vi "Define Advanced Sequence.vi"(4 "Current Level Start":dbl, 5 "name":string, 6 "Current Level Stop":dbl, 7 "Voltage Level Stop":dbl, 8 "error in (no error)":errorcluster, 9 "Points per Output Function":i32, 10 "Voltage Level Start":dbl, 11 "IVI Refnum in":refnum<k15>) -> (0 "error out":errorcluster, 1 "sequence name":string, 2 "Numeric":i32, 3 "IVI Refnum out":refnum<k15>)   [LabVIEW 2020]
uses:
  <instrlib>/niDCPower/nidcpower.llb/niDCPower Sequence Attribute Type.ctl
  <instrlib>/niDCPower/nidcpower.llb/niDCPower Output Function.ctl
  <instrlib>/niDCPower/nidcpower.llb/niDCPower Create Advanced Sequence Step With Channels.vi
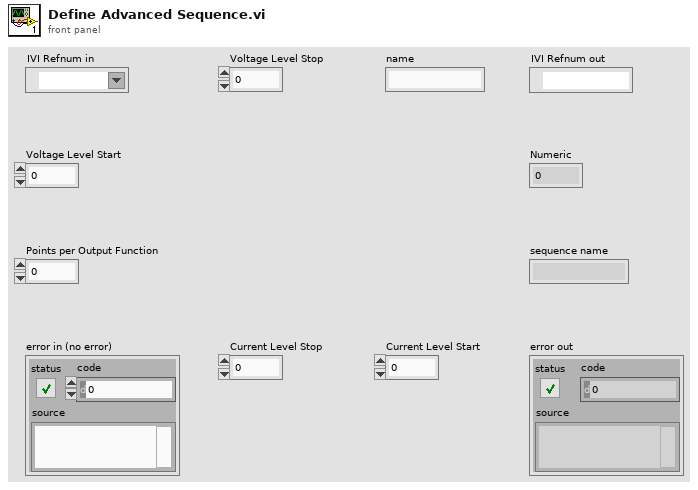
[diagram p1: front panel]
types:
  T1 = typedef "niDCPower Sequence Attribute Type.ctl" = i32
  T2 = typedef "niDCPower Output Function.ctl" = i32
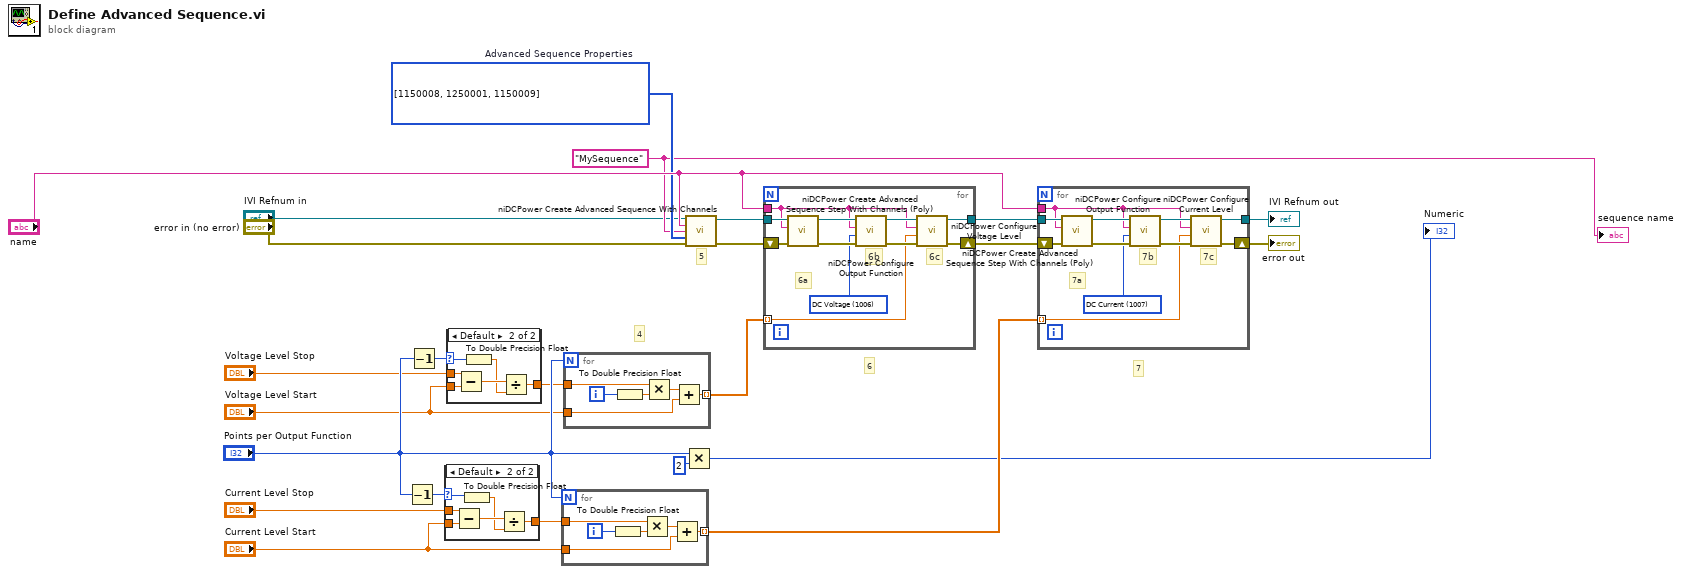
[diagram p0: block diagram]
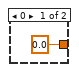
[diagram p2: hidden frame]
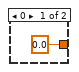
[diagram p3: hidden frame]
diagram:
  w23 = T1[] [1150008, 1250001, 1150009] items=["Source -> Output Function"=1150008, "Source -> Output Enabled"=1250006, "Source -> Output Resistance"=1150061, "Source -> Transient Response"=1150062, "Source -> Custom Transient Response -> Voltage Gain Bandwidth"=1150067, "Source -> Custom Transient Response -> Voltage Compensation Frequency"=1150068, "Source -> Custom Transient Response -> Voltage Pole-Zero Ratio"=1150069, "Source -> Custom Transient Response -> Current Gain Bandwidth"=1150070, "Source -> Custom Transient Response -> Current Compensation Frequency"=1150071, "Source -> Custom Transient Response -> Current Pole-Zero Ratio"=1150072, "Source -> DC Voltage -> Voltage Level"=1250001, "Source -> DC Voltage -> Voltage Level Range"=1150005, "Source -> DC Voltage -> Current Limit"=1250005, "Source -> DC Voltage -> Current Limit High"=1150187, "Source -> DC Voltage -> Current Limit Low"=1150188, "Source -> DC Voltage -> Current Limit Range"=1150004, "Source -> DC Current -> Current Level"=1150009, "Source -> DC Current -> Current Level Range"=1150011, "Source -> DC Current -> Voltage Limit"=1150010, "Source -> DC Current -> Voltage Limit High"=1150185, "Source -> DC Current -> Voltage Limit Low"=1150186, "Source -> DC Current -> Voltage Limit Range"=1150012, "Source -> DC Current -> Current Level Slew Rate -> Rising"=1150343, "Source -> DC Current -> Current Level Slew Rate -> Falling"=1150344, "Source -> Pulse Voltage -> Pulse Voltage Level"=1150080, "Source -> Pulse Voltage -> Pulse Bias Voltage Level"=1150082, "Source -> Pulse Voltage -> Pulse Voltage Level Range"=1150084, "Source -> Pulse Voltage -> Pulse Current Limit"=1150081, "Source -> Pulse Voltage -> Pulse Current Limit High"=1150193, "Source -> Pulse Voltage -> Pulse Current Limit Low"=1150194, "Source -> Pulse Voltage -> Pulse Bias Current Limit"=1150083, "Source -> Pulse Voltage -> Pulse Bias Current Limit High"=1150195, "Source -> Pulse Voltage -> Pulse Bias Current Limit Low"=1150196, "Source -> Pulse Voltage -> Pulse Current Limit Range"=1150085, "Source -> Pulse Current -> Pulse Current Level"=1150086, "Source -> Pulse Current -> Pulse Bias Current Level"=1150088, "Source -> Pulse Current -> Pulse Current Level Range"=1150090, "Source -> Pulse Current -> Pulse Voltage Limit"=1150087, "Source -> Pulse Current -> Pulse Voltage Limit High"=1150189, "Source -> Pulse Current -> Pulse Voltage Limit Low"=1150190, "Source -> Pulse Current -> Pulse Bias Voltage Limit"=1150089, "Source -> Pulse Current -> Pulse Bias Voltage Limit High"=1150191, "Source -> Pulse Current -> Pulse Bias Voltage Limit Low"=1150192, "Source -> Pulse Current -> Pulse Voltage Limit Range"=1150091, "Source -> Advanced -> Source Delay"=1150051, "Source -> Advanced -> Pulse Bias Delay"=1150092, "Source -> Advanced -> Pulse On Time"=1150093, "Source -> Advanced -> Pulse Off Time"=1150094, "Source -> Advanced -> OVP Enabled"=1250002, "Source -> Advanced -> OVP Limit"=1250003, "Source -> Advanced -> Compliance Limit Symmetry"=1150184, "Source -> Advanced -> Sequence Step Delta Time"=1150198, "Source -> Advanced -> Conduction Voltage -> Mode"=1150350, "Source -> Advanced -> Conduction Voltage -> On Threshold"=1150351, "Source -> Advanced -> Conduction Voltage -> Off Threshold"=1150352, "Measurement -> Sense"=1150013, "Measurement -> Aperture Time"=1150058, "Measurement -> Measure Record Length"=1150063, "Measurement -> Advanced -> DC Noise Rejection"=1150066, "Measurement -> Autorange"=1150244, "Measurement -> Advanced -> Autorange Behavior"=1150245, "Measurement -> Advanced -> Autorange Aperture Time Mode"=1150246, "Measurement -> Advanced -> Autorange Minimum Aperture Time"=1150247, "Measurement -> Advanced -> Autorange Minimum Aperture Time Units"=1150248, "Measurement -> Advanced -> Autorange Minimum Current Range"=1150255, "Measurement -> Advanced -> Autorange Minimum Voltage Range"=1150256, "Measurement -> Advanced -> Autorange Threshold Mode"=1150257, "Measurement -> Advanced -> Autorange Maximum Delay After Range Change"=1150322, "LCR -> Instrument Mode"=1150208, "LCR -> Source Delay Mode"=1150315, "LCR -> Measurement Time"=1150218, "LCR -> Custom Measurement Time"=1150258, "LCR -> AC Stimulus -> Function"=1150209, "LCR -> AC Stimulus -> Frequency"=1150210, "LCR -> AC Stimulus -> Voltage Amplitude"=1150211, "LCR -> AC Stimulus -> Current Amplitude"=1150212, "LCR -> AC Stimulus -> Advanced -> Voltage Range"=1150265, "LCR -> AC Stimulus -> Advanced -> Current Range"=1150267, "LCR -> AC Stimulus -> Advanced -> Source Aperture Time"=1150349, "LCR -> DC Bias -> Source"=1150213, "LCR -> DC Bias -> Voltage Level"=1150214, "LCR -> DC Bias -> Current Level"=1150215, "LCR -> DC Bias -> Advanced -> Voltage Range"=1150266, "LCR -> DC Bias -> Advanced -> Current Range"=1150274, "LCR -> DC Bias -> Advanced -> Transient Response"=1150347, "LCR -> Compensation -> Open -> Enabled"=1150220, "LCR -> Compensation -> Open -> Conductance"=1150261, "LCR -> Compensation -> Open -> Susceptance"=1150262, "LCR -> Compensation -> Short -> Enabled"=1150221, "LCR -> Compensation -> Short -> Resistance"=1150263, "LCR -> Compensation -> Short -> Reactance"=1150264, "LCR -> Compensation -> Load -> Enabled"=1150222, "LCR -> Compensation -> Load -> Measured Resistance"=1150268, "LCR -> Compensation -> Load -> Measured Reactance"=1150269, "LCR -> Compensation -> Load -> Actual Resistance"=1150270, "LCR -> Compensation -> Load -> Actual Reactance"=1150271, "LCR -> Impedance Range -> Impedance Range"=1150217, "LCR -> Impedance Range -> Impedance Autorange"=1150216, "LCR -> Impedance Range -> Advanced -> Impedance Range Source"=1150321, "LCR -> Impedance Range -> Advanced -> Load Resistance"=1150318, "LCR -> Impedance Range -> Advanced -> Load Inductance"=1150319, "LCR -> Impedance Range -> Advanced -> Load Capacitance"=1150320]  # Advanced Sequence Properties
  w13 = "MySequence" ("sequence name")
  # "4"
  # "7"
  # "6"
  # "5"
  n1 = Decrement(x="Points per Output Function") -> (x-1=w9:i32)
  n2 = Decrement(x="Points per Output Function") -> (x-1=w4:i32)
  n3 = case shown="Default" w9 {
    selector: w9 -> [_ w26]
    tunnel: "Current Level Stop" -> [_ w31]
    tunnel: [0.0 w29] -> w8
    tunnel: "Current Level Start" -> [_ w27]
    frame 0 {
    }
    frame Default {
      n4 = Subtract(x=w31, y=w27) -> (x-y=w30:dbl)
      n5 = To Double Precision Float(number=w26) -> (double precision float=w28:dbl)
      n6 = Divide(x=w30, y=w28) -> (x/y=w29:dbl)
    }
  }
  n7 = case shown="Default" w4 {
    selector: w4 -> [_ w33]
    tunnel: "Voltage Level Stop" -> [_ w38]
    tunnel: [0.0 w36] -> w5
    tunnel: "Voltage Level Start" -> [_ w34]
    frame 0 {
    }
    frame Default {
      n8 = Subtract(x=w38, y=w34) -> (x-y=w37:dbl)
      n9 = To Double Precision Float(number=w33) -> (double precision float=w35:dbl)
      n10 = Divide(x=w37, y=w35) -> (x/y=w36:dbl)
    }
  }
  n11 = for {
    N: "Points per Output Function" -> [_]
    tunnel: w8 -> [w44]
    tunnel: "Current Level Start" -> [w41]
    tunnel: [w39] -> w22 mode=indexing
    i -> [w43]
    n12 = To Double Precision Float(number=w43) -> (double precision float=w40:dbl)
    n13 = Multiply(x=w44, y=w40) -> (x*y=w42:dbl)
    n14 = Add(x=w42, y=w41) -> (x+y=w39:dbl)
  }
  n15 = for {
    N: "Points per Output Function" -> [_]
    tunnel: w5 -> [w50]
    tunnel: "Voltage Level Start" -> [w47]
    tunnel: [w45] -> w14 mode=indexing
    i -> [w49]
    n16 = To Double Precision Float(number=w49) -> (double precision float=w46:dbl)
    n17 = Multiply(x=w50, y=w46) -> (x*y=w48:dbl)
    n18 = Add(x=w48, y=w47) -> (x+y=w45:dbl)
  }
  n19 = Multiply(x="Points per Output Function", y=2) -> (x*y=→"Numeric":i32)
  n20 = call <instrlib>:"niDCPower Create Advanced Sequence With Channels.vi"("instrument handle"="IVI Refnum in", "channel name"="name", "sequence name"=w13, "advanced sequence properties"=w23, "error in (no error)"="error in (no error)") -> ("instrument handle out"=w12:refnum<k15>, "error out"=w11:errorcluster)  [unwired: 9 in]
  n21 = for {
    tunnel: w12 -> [w60]
    tunnel: [w55] -> w18
    shift-right: [w54] -> w19
    shift-left: w11 -> [w61]
    tunnel: w14 -> [w52] mode=indexing
    tunnel: "name" -> [w51]
    w53 = T2 1006 items=["DC Voltage"=1006, "DC Current"=1007, "Pulse Voltage"=1049, "Pulse Current"=1050] ("output function")
    # "6c"
    # "6b"
    # "6a"
    n22 = call-poly <instrlib>:"niDCPower Create Advanced Sequence Step With Channels (Poly).vi"("error in (no error)"=w61, "channel name"=w51, "instrument handle"=w60) -> ("error out"=w58:errorcluster, "instrument handle out"=w59:refnum<k15>)  [unwired: 7 in]
    n23 = call <instrlib>:"niDCPower Configure Output Function.vi"("error in (no error)"=w58, "output function"=w53, "channel name"=w51, "instrument handle"=w59) -> ("error out"=w56:errorcluster, "instrument handle out"=w57:refnum<k15>)  [unwired: 6 in]
    n24 = call <instrlib>:"niDCPower Configure Voltage Level.vi"("error in (no error)"=w56, "voltage level"=w52, "channel name"=w51, "instrument handle"=w57) -> ("error out"=w54:errorcluster, "instrument handle out"=w55:refnum<k15>)  [unwired: 6 in]
  }
  n25 = for {
    tunnel: w18 -> [w71]
    tunnel: [w66] -> w21
    shift-right: [w65] -> w20
    shift-left: w19 -> [w72]
    tunnel: w22 -> [w63] mode=indexing
    tunnel: "name" -> [w62]
    w64 = T2 1007 items=["DC Voltage"=1006, "DC Current"=1007, "Pulse Voltage"=1049, "Pulse Current"=1050] ("output function")
    # "7c"
    # "7b"
    # "7a"
    n26 = call-poly <instrlib>:"niDCPower Create Advanced Sequence Step With Channels (Poly).vi"("error in (no error)"=w72, "channel name"=w62, "instrument handle"=w71) -> ("error out"=w69:errorcluster, "instrument handle out"=w70:refnum<k15>)  [unwired: 7 in]
    n27 = call <instrlib>:"niDCPower Configure Output Function.vi"("error in (no error)"=w69, "output function"=w64, "channel name"=w62, "instrument handle"=w70) -> ("error out"=w67:errorcluster, "instrument handle out"=w68:refnum<k15>)  [unwired: 6 in]
    n28 = call <instrlib>:"niDCPower Configure Current Level.vi"("error in (no error)"=w67, "current level"=w63, "channel name"=w62, "instrument handle"=w68) -> ("error out"=w65:errorcluster, "instrument handle out"=w66:refnum<k15>)  [unwired: 6 in]
  }
  "IVI Refnum out" <- w21
  "error out" <- w20
  "sequence name" <- w13
